vi "EvaluatePoint.vi"(8 "error in (no error)":errorcluster, 9 "Game":refnum<class "Game.lvclass">, 10 "Point":dbl[](array[numeric]), 11 "Evaluator in":refnum<class "Evaluator.lvclass">) -> (0 "error out":errorcluster, 2 "Evaluation":dbl, 3 "Evaluator out":refnum<class "Evaluator.lvclass">)   [LabVIEW 2023, in "Evaluator.lvclass"]
uses:
  Evaluator.lvclass
  Game_class/Game.lvclass
  Evaluator.lvclass/Evaluator.ctl
  Criteria/Criterion_class/Criterion.lvclass
  Utilities_class/Utilities.lvclass
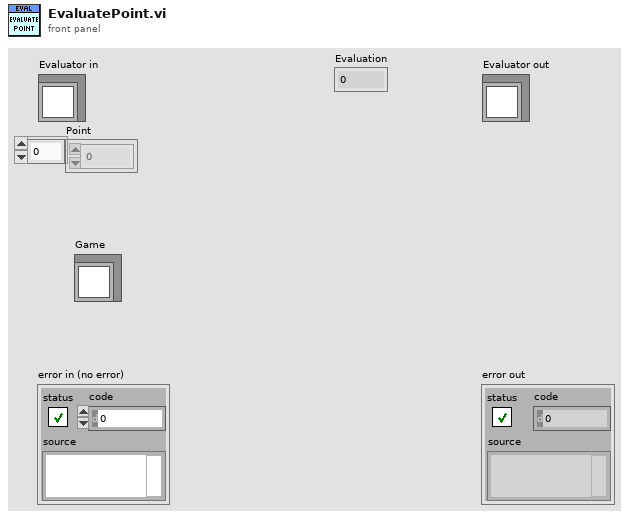
[diagram p1: front panel]
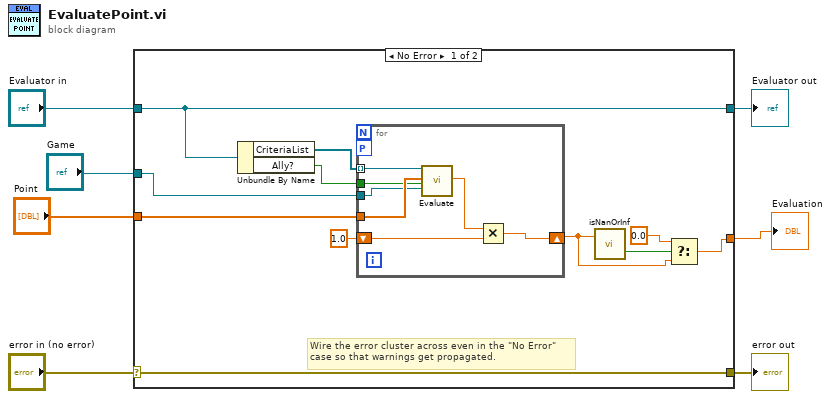
[diagram p0: block diagram]
diagram:
  n1 = case shown="No Error" "error in (no error)" {
    selector: "error in (no error)" -> [w18 w27]
    tunnel: [w18 w27] -> w6
    tunnel: [w17 w26] -> w4
    tunnel: "Evaluator in" -> [w17 w26]
    tunnel: "Point" -> [w15 _]
    tunnel: [w12 _] -> w2
    tunnel: "Game" -> [w8 _]
    frame No Error {
      # "Wire the error cluster across even in the \"No Error\"\ncase so that warnings get propagated."
      n2 = Unbundle By Name(w17) -> ("CriteriaList"=w16:refnum<class "Criterion.lvclass">[], "Ally?"=w14:bool)
      n3 = for {
        tunnel: w16 -> [w20] mode=indexing
        tunnel: w15 -> [w25]
        tunnel: w14 -> [w24]
        shift-right: [w21] -> w9
        shift-left: 1.0 -> [w22]
        tunnel: w8 -> [w19]
        workers-P: _ -> [_]
        n4 = call-dynamic "Evaluate.vi"("object in"=w20, "Point"=w25, "Ally?"=w24, "Game"=w19) -> ("Evaluation"=w23:dbl)  [unwired: 13 in, 2 out]
        n5 = Multiply(x=w23, y=w22) -> (x*y=w21:dbl)
      }
      n6 = call "isNanOrInf.vi"("value"=w9) -> ("narOrInf?"=w11:bool)  [unwired: 13 in, 5 out]
      n7 = Select(t=0.0, s=w11, f=w9) -> (s? t:f=w12:dbl)
    }
    frame Error {
    }
  }
  "error out" <- w6
  "Evaluator out" <- w4
  "Evaluation" <- w2
